vi "createCmdQueue.vi"(8 "error in (no error)":errorcluster, 11 "tcpServer in":refnum<class "TcpServer.lvclass">) -> (0 "error out":errorcluster, 3 "tcpServer out":refnum<class "TcpServer.lvclass">)   [LabVIEW 2018, in "TcpServer.lvclass"]
doc: "Create command queue reference."
uses:
  TcpServer.lvclass
  TcpServer.lvclass/TcpServer.ctl
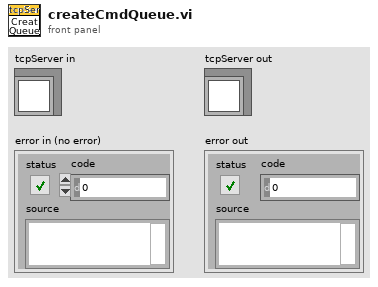
[diagram p1: front panel]
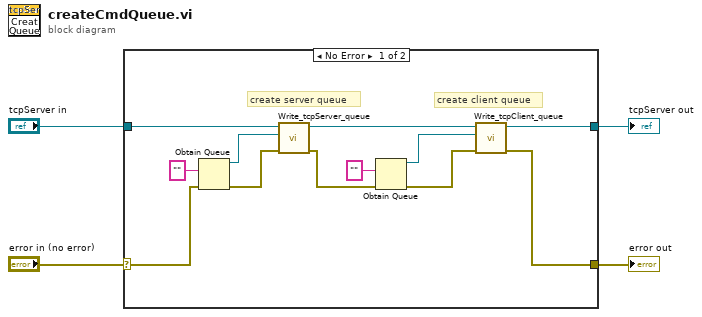
[diagram p0: block diagram]
diagram:
  n1 = case shown="No Error" "error in (no error)" {
    selector: "error in (no error)" -> [w9 w18]
    tunnel: "tcpServer in" -> [w16 w17]
    tunnel: [w11 w17] -> w3
    tunnel: [w5 w18] -> w1
    frame No Error {
      # "create client queue"
      # "create server queue"
      n2 = Obtain Queue(element data type="", error in (no error)=w9) -> (queue out=w15:refnum<queue>, error out=w8:errorcluster)  [unwired: 3 in, 1 out]
      n3 = call "Write_tcpServer_queue.vi"("error in (no error)"=w8, "tcpServer queue"=w15, "tcpServer in"=w16) -> ("error out"=w7:errorcluster, "tcpServer out"=w12:refnum<class "TcpServer.lvclass">)  [unwired: 7 in]
      n4 = Obtain Queue(element data type="", error in (no error)=w7) -> (queue out=w10:refnum<queue>, error out=w6:errorcluster)  [unwired: 3 in, 1 out]
      n5 = call "Write_tcpClient_queue.vi"("error in (no error)"=w6, "tcpClient queue"=w10, "tcpServer in"=w12) -> ("error out"=w5:errorcluster, "tcpServer out"=w11:refnum<class "TcpServer.lvclass">)  [unwired: 7 in]
    }
    frame Error {
    }
  }
  "error out" <- w1
  "tcpServer out" <- w3
